vi "test_timer.vi"() -> ()   [LabVIEW 2009]
uses:
  modules/timer/tlc_timer_Command_enum.ctl
panel:
  out "Elapsed":bool
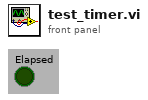
[diagram p1: front panel]
types:
  T1 = typedef "tlc_timer_Command_enum.ctl" = enum16{"Start Timer", "Check Timer"}
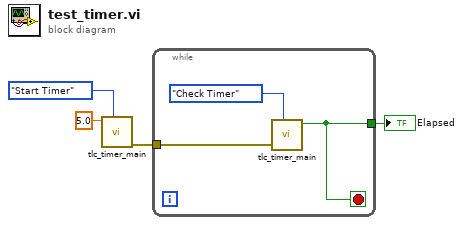
[diagram p0: block diagram]
diagram:
  n1 = call "tlc_timer_main.vi"("Command (Check Timer)"=tlc_timer_Command_enum."Start Timer", "Target Time (s)"=5.0) -> ("error out"=w3:errorcluster)  [unwired: 8 in, 1 out]
  n2 = while {
    tunnel: w3 -> [w6]
    tunnel: [w5] -> w2
    stop <- w5 stop-if-true
    n3 = call "tlc_timer_main.vi"("Command (Check Timer)"=tlc_timer_Command_enum."Check Timer", "error in (no error)"=w6) -> ("Elapsed"=w5:bool)  [unwired: 8 in, 1 out]
  }
  "Elapsed" <- w2
